vi "MCP4725_with_GraphforLoopSingleArduino.vi"() -> ()   [LabVIEW 2017]
uses:
  <vilib>/MakerHub/LINX/Public/Peripherals/Analog/Analog Read N Chans.vi
  <vilib>/MakerHub/LINX/Private/Local IO/LinxI2cWrite.vi
  <vilib>/MakerHub/LINX/Public/Utilities/Check Channel.vi
  <vilib>/MakerHub/LINX/Private/Local IO/LinxAnalogRead.vi
  <vilib>/MakerHub/LINX/Public/Utilities/Open Serial.vi
  <vilib>/MakerHub/LINX/Private/Utilties/Generate Error.vi
  <vilib>/Utility/file.llb/Write Delimited Spreadsheet (DBL).vi
  <vilib>/MakerHub/LINX/LMH-LINX.lvlib
panel:
  in  "Save Data":bool
  out "XY Graph 2":cluster{dbl[], dbl[]}[](graph)
  out "XY Graph":cluster{dbl[], dbl[]}(graph)
  out "Voltage on Analog Channel":dbl(knob) scale=0.0..75.0
  out "Current Value written to \nDAC  input":u16
  out "Device Name":string
  out "Error Out":errorcluster
  in  "Data Collection\nTime  Interval (ms)":u32
  in  "Arduino \nSerial Port":refnum<visa-resource-name>="N/A"
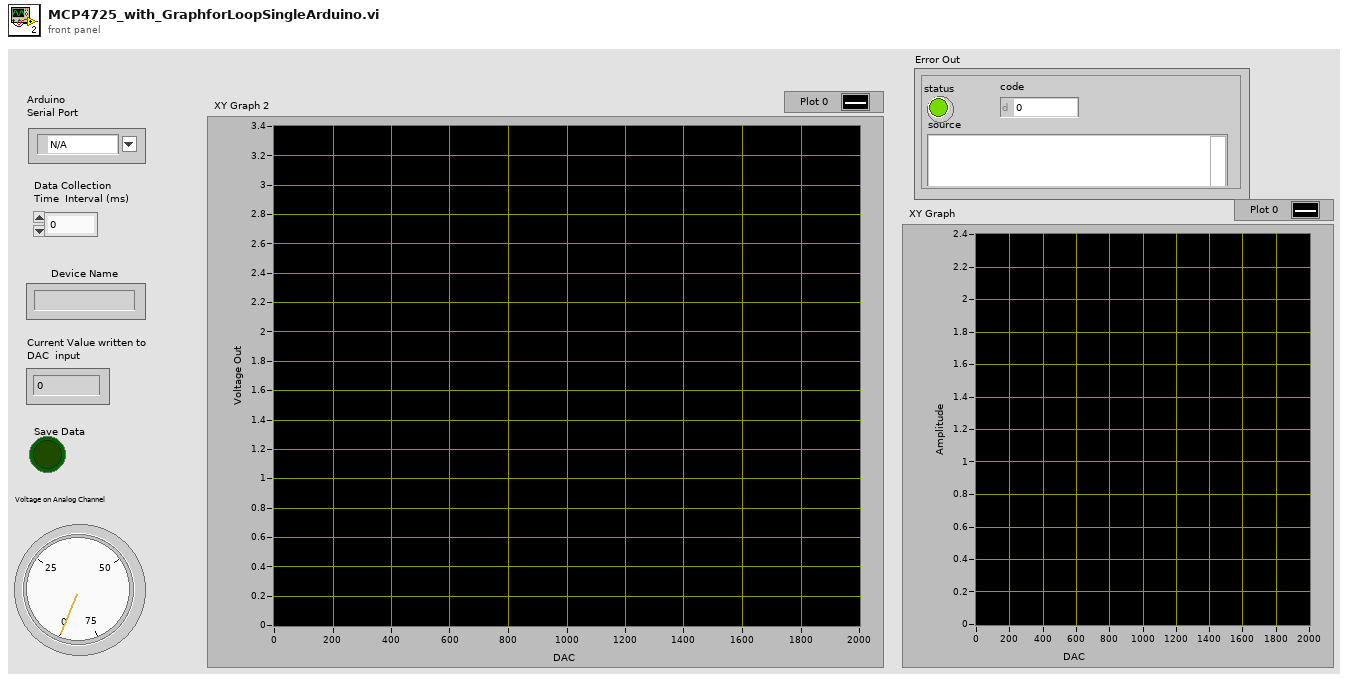
[diagram p1: front panel]
types:
  T1 = typedef "LMH-LINX.lvlib/LINX Ref.ctl" = cluster{"IO":T2, "Interface":T3, "LINX Device Config":T4}
  T2 = typedef "LMH-LINX.lvlib/Platform.ctl" = enum16{"Remote", "Local"}
  T3 = typedef "LMH-LINX.lvlib/Interface.ctl" = enum16{"Serial", "TCP"}
  T4 = typedef "LMH-LINX.lvlib/Device.lvlib/LINX Device Config.ctl" = cluster{"Interface":T3, "COM Port":refnum<visa-resource-name>, "TCP Configuration":T5, "Device Family":u8, "Device ID":u8, "Device Name":string, "TCP Ref":refnum<k5>, "Channels":T6}
  T5 = typedef "LMH-LINX.lvlib/Device.lvlib/TCP Config.ctl" = cluster{"IP Address":string, "Port":u16}
  T6 = typedef "LMH-LINX.lvlib/Channels.ctl" = cluster{"DI":u8[], "DO":u8[], "AI":u8[], "AO":u8[], "PWM":u8[], "QE":u8[], "UART":u8[], "I2C 2":u8[], "SPI":u8[], "CAN":u8[], "Servo":u8[], "AI Ref (V)":dbl, "AI Resolution (Bits)":u8, "AO Ref (V)":dbl, "AO Resolution (Bits)":u8}
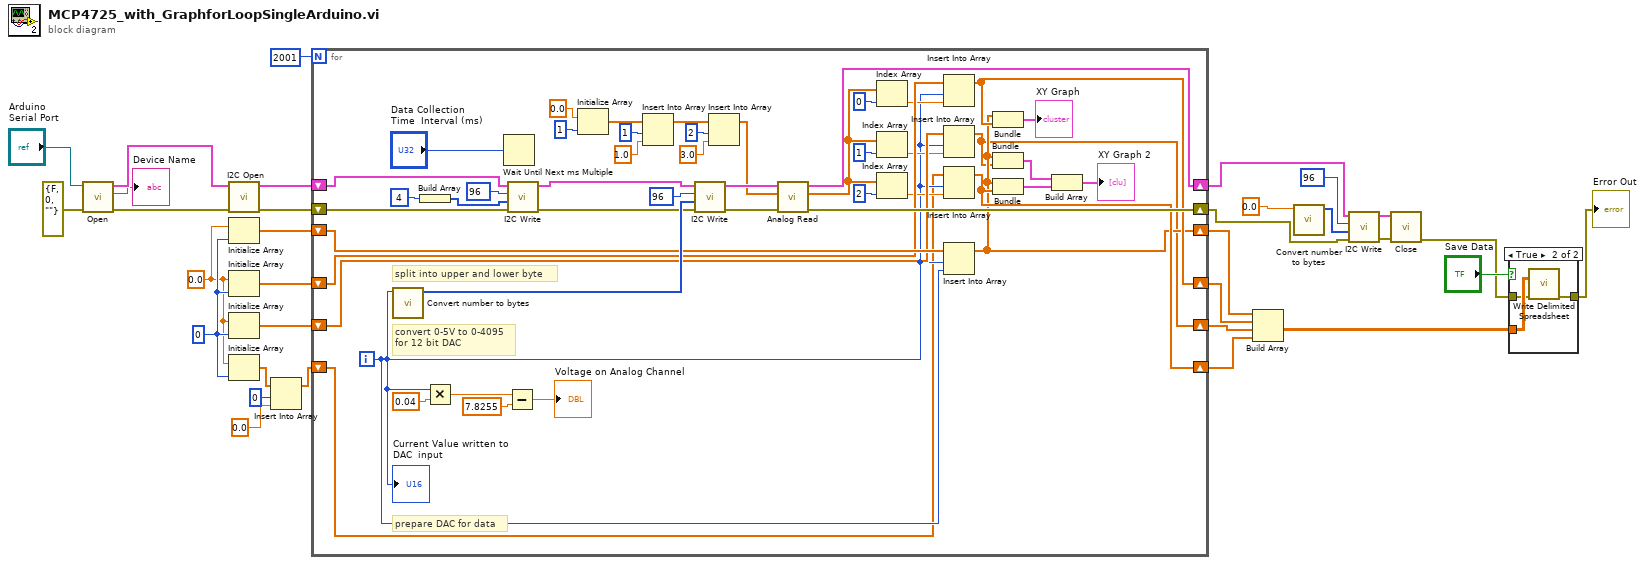
[diagram p0: block diagram]
diagram:
  w16 = 0.0 ("element")
  w17 = 0 ("dimension size")
  n1 = call-poly <vilib>:"Open.vi"("Error In"=errorcluster {"status"=FALSE, "code"=0, "source"=""}, "Serial Port"="Arduino \nSerial Port") -> ("Error Out"=w30:errorcluster, "Device Name"=→"Device Name":string, "LINX Resource"=w31:T1)  [unwired: 7 in]
  n2 = call <vilib>:"I2C Open.vi"("Error In"=w30, "LINX Resource"=w31) -> ("Error Out"=w27:errorcluster, "LINX Resource"=w28:T1)  [unwired: 8 in]
  n3 = Initialize Array(w16, w17) -> (w25:dbl[])
  n4 = Initialize Array(w16, w17) -> (w24:dbl[])
  n5 = Initialize Array(w16, w17) -> (w15:dbl[])
  n6 = Initialize Array(w16, w17) -> (w4:dbl[])
  n7 = Insert Into Array(array=w4, index=0, new element=0.0 ("new element/subarray")) -> (w1:dbl[])
  n8 = for {
    N: 2001 -> [_]
    shift-right: [w70] -> w10
    shift-left: w28 -> [w79]
    shift-right: [w68] -> w7
    shift-left: w27 -> [w78]
    shift-right: [w42] -> w14
    shift-left: w25 -> [w66]
    shift-right: [w49] -> w13
    shift-left: w24 -> [w65]
    shift-right: [w41] -> w12
    shift-left: w15 -> [w48]
    shift-right: [w43] -> w11
    shift-left: w1 -> [w33]
    i -> [w37]
    # "prepare DAC for data"
    # "convert 0-5V to 0-4095\nfor 12 bit DAC"
    # "split into upper and lower byte"
    n9 = call "Convert number to bytes.vi"("Numeric"=w37) -> ("Array"=w76:u8[])  [unwired: 10 in]
    n10 = Build Array(u8 4) -> (w72:u8[])
    n11 = Multiply(x=w37, y=0.04) -> (x*y=w52:dbl)
    n12 = Wait Until Next ms Multiple(millisecond multiple="Data Collection\nTime  Interval (ms)") -> ()  [unwired: 1 out]
    n13 = Subtract(x=w52, y=7.8255) -> (x-y=→"Voltage on Analog Channel":dbl)
    n14 = call <vilib>:"I2C Write.vi"("Error In"=w78, "Data"=w72, "I2C Slave Address (0)"=u8 96, "LINX Resource"=w79) -> ("Error Out"=w63:errorcluster, "LINX Resource"=w62:T1)  [unwired: 6 in]
    n15 = Initialize Array(0.0 ("element"), 1 ("dimension size")) -> (w59:dbl[])
    n16 = Insert Into Array(array=w59, index=1, new element=1.0 ("new element/subarray")) -> (w56:dbl[])
    n17 = call <vilib>:"I2C Write.vi"("Error In"=w63, "Data"=w76, "I2C Slave Address (0)"=u8 96, "LINX Resource"=w62) -> ("Error Out"=w69:errorcluster, "LINX Resource"=w71:T1)  [unwired: 6 in]
    n18 = Insert Into Array(array=w56, index=2, new element=3.0 ("new element/subarray")) -> (w53:dbl[])
    n19 = call-poly <vilib>:"Analog Read.vi"("Error In"=w69, "AI Channel(s)"=w53, "LINX Resource"=w71) -> ("Error Out"=w68:errorcluster, "Voltages"=w45:dbl[], "LINX Resource"=w70:T1)  [unwired: 5 in, 1 out]
    n20 = Index Array(array=w45, index=0) -> (element=w44:dbl)
    n21 = Index Array(array=w45, index=1) -> (element=w47:dbl)
    n22 = Index Array(array=w45, index=2) -> (element=w46:dbl)
    n23 = Insert Into Array(array=w65, index=w37, new element=w44) -> (w49:dbl[])
    n24 = Insert Into Array(array=w48, index=w37, new element=w47) -> (w41:dbl[])
    n25 = Insert Into Array(array=w33, index=w37, new element=w46) -> (w43:dbl[])
    n26 = Insert Into Array(array=w66, index=w37, new element=w37) -> (w42:dbl[])
    n27 = Bundle(w42, w49) -> (→"XY Graph":cluster{dbl[], dbl[]})  [unwired: 1 in]
    n28 = Bundle(w42, w41) -> (w39:cluster{dbl[], dbl[]})  [unwired: 1 in]
    n29 = Bundle(w42, w43) -> (w40:cluster{dbl[], dbl[]})  [unwired: 1 in]
    n30 = Build Array(w39, w40) -> (→"XY Graph 2":cluster{dbl[], dbl[]}[])
    "Current Value written to \nDAC  input" <- w37
  }
  n31 = Build Array(w14, w13, w12, w11) -> (w9:dbl[][])
  n32 = call "Convert number to bytes.vi"("Numeric"=0.0) -> ("Array"=w21:u8[])  [unwired: 10 in]
  n33 = call <vilib>:"I2C Write.vi"("Error In"=w7, "Data"=w21, "I2C Slave Address (0)"=u8 96, "LINX Resource"=w10) -> ("Error Out"=w20:errorcluster, "LINX Resource"=w19:T1)  [unwired: 6 in]
  n34 = call <vilib>:"Close.vi"("Error In"=w20, "LINX Resource"=w19) -> ("Error Out"=w6:errorcluster)  [unwired: 9 in]
  n35 = case shown="True" "Save Data" {
    tunnel: [w80 w83] -> w5
    tunnel: w6 -> [w80 w81]
    tunnel: w9 -> [_ w82]
    frame False {
    }
    frame True {
      n36 = call-poly <vilib>:"Write Delimited Spreadsheet.vi"("2D data"=w82, "error in (no error)"=w81) -> ("error out"=w83:errorcluster)  [unwired: 12 in, 1 out]
    }
  }
  "Error Out" <- w5
